vi "PID_control_main.vi"() -> ()   [LabVIEW 2019]
doc: "This example demonstrates how to simulate a general PID controller."
uses:
  <vilib>/addons/control/pid/pid.llb/PID (DBL).vi
  <vilib>/addons/control/pid/NI_PID_pid.lvlib
panel:
  in  "P_init":dbl=4.5 caption="psi" format="%#_13g"
  in  "dt":dbl=100.0 caption="sec"
  out "F_O":dbl=100.0 caption="L/m"
  in  "V":dbl=1000.0 caption="L"
  in  "F_I":dbl=100.0 caption="L/m"
  out "Manipulated variable":dbl(graph)
  in  "P_set":dbl(slide)=4.0 min=0.0 max=0.0 scale=0.0..100.0
  out "MV:":dbl(slide)=18.78965245852964 scale=-100.0..100.0
  out "P_read":dbl(slide)=60.754431603254424 scale=0.0..100.0
  in  "PID gains":T1={"proportional gain (Kc)"=20.0, "integral time (Ti, min)"=0.008, "derivative time (Td, min)"=0.001} {"derivative time (Td, min)" format="%.3f"; "integral time (Ti, min)" format="%.3f"; "proportional gain (Kc)" format="%.3f"}
  in  "Stop":bool
  out "Process variable and Setpoint":cluster{"initial PV":dbl, "SP:":dbl}(graph)
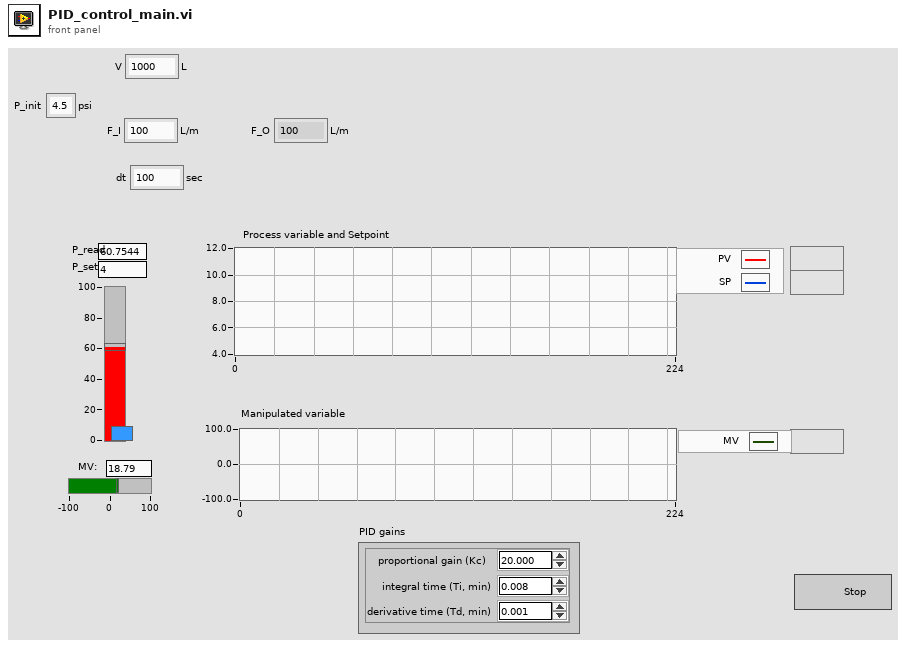
[diagram p1: front panel]
types:
  T1 = cluster{"proportional gain (Kc)":dbl, "integral time (Ti, min)":dbl, "derivative time (Td, min)":dbl}
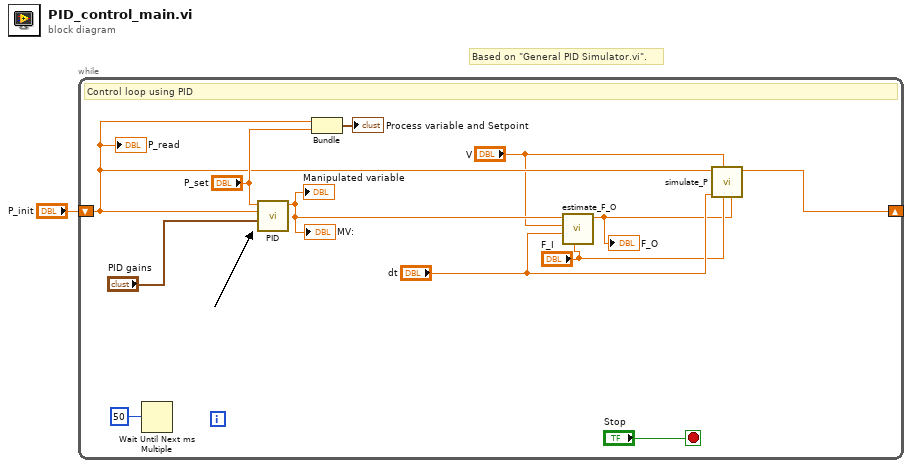
[diagram p0: block diagram]
diagram:
  # "Based on \"General PID Simulator.vi\"."
  n1 = while {
    shift-left: "P_init" -> [w7]
    shift-right: [w2] -> _
    stop <- "Stop" stop-if-true
    # "Control loop using PID"
    n2 = Wait Until Next ms Multiple(millisecond multiple=u32 50 ("unsigned 32bit integer")) -> ()  [unwired: 1 out]
    n3 = call-poly <vilib>:"PID.vi"("PID gains"="PID gains", "process variable"=w7, "setpoint"="P_set") -> ("output"=w8:dbl)  [unwired: 7 in, 1 out]
    "MV:" <- w8
    "Manipulated variable" <- w8
    n4 = Bundle("P_init"=w7, "P_set"="P_set") -> (→"Process variable and Setpoint":cluster{"P_init":dbl, "P_set":dbl})  [unwired: 1 in]
    n5 = call "estimate_F_O.vi"("F_I"="F_I", "dt"="dt", "V"="V", "P_change"=w8) -> ("F_O"=w3:dbl)  [unwired: 7 in]
    "F_O" <- w3
    n6 = call "simulate_P.vi"("F_O"=w3, "F_I"="F_I", "V"="V", "dt"="dt", "P_in"=w7) -> ("P_out"=w2:dbl)  [unwired: 6 in]
    "P_read" <- w7
  }
